vi "test Add-Find-Remove Custom Device.vi"(8 "error in":errorcluster, 11 "TestCase in":refnum<class "Scripting.lvclass">) -> (0 "error out":errorcluster, 3 "TestCase out":refnum<class "Scripting.lvclass">)   [LabVIEW 2020, in "Scripting.lvclass"]
uses:
  Scripting.lvclass
  C:/dev/git/niveristand-custom-device-testing-tools/VeriStandScriptingTestCase/VeriStandScriptingTestCase.lvclass
  niveristand-custom-device-testing-tools/VeriStandScriptingTestCase/VeriStandScriptingTestCase.lvclass/VeriStandScriptingTestCase.ctl
  niveristand-custom-device-testing-tools/VeriStandScriptingTestCase/Read Target.vi
  NationalInstruments.VeriStand.SystemDefinitionAPI
  <vilib>/addons/_JKI Toolkits/VI Tester/TestCase.llb/TestCase.lvclass
  Scripting/AIM MIL-STD-1553 Scripting.lvlib
  C:/Program Files (x86)/National Instruments/LabVIEW 2020/vi.lib/addons/_JKI Toolkits/VI Tester/TestCase.llb/TestCase.lvclass
  C:/dev/git/niveristand-aim-milStd1553-custom-device/Source/Custom Device Support/Tests/Unit/Scripting/Scripting.lvclass
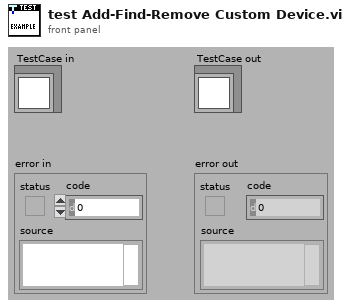
[diagram p1: front panel]
types:
  T1 = typedef "Custom Device API.lvlib/Custom Device Item Ref.ctl" = u64
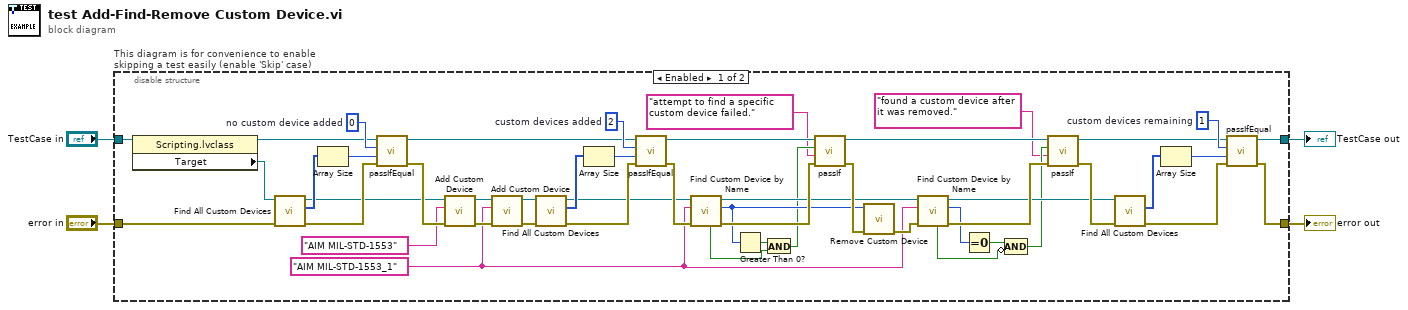
[diagram p0: block diagram]
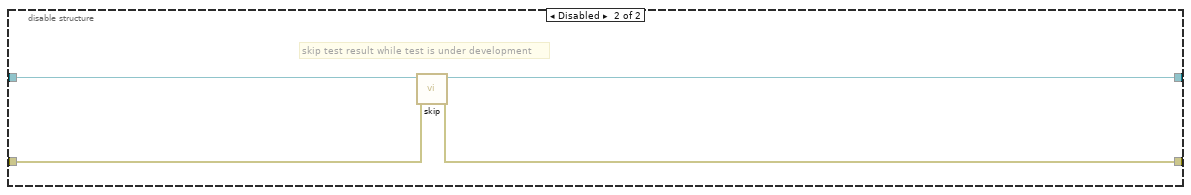
[diagram p2: hidden frame]
diagram:
  n1 = disable-structure "This diagram is for convenience to enable skipping a test easily (enable 'Skip' case)" shown="Enabled" {
    disable-tunnel: "TestCase in" -> [w20 w57]
    disable-tunnel: [w23 w55] -> w1
    disable-tunnel: [w22 w56] -> w3
    disable-tunnel: "error in" -> [w53 w54]
    frame Enabled {
      w7 = "AIM MIL-STD-1553_1" ("name")
      w27 = 1  # custom devices remaining
      w43 = 2  # custom devices added
      w50 = 0  # no custom device added
      n2 = property class="Scripting.lvclass"(reference=w20) -> (reference out=w18:refnum<class "Scripting.lvclass">, "Target"=w19:refnum<k24>)  [unwired: 1 in, 1 out]
      n3 = call "Find All Custom Devices.vi"("error in"=w53, "target"=w19) -> ("error out"=w49:errorcluster, "custom device refs"=w52:T1[], "target out"=w47:refnum<k24>)  [unwired: 7 in]
      n4 = Array Size(array=w52) -> (size(s)=w51:i32)
      n5 = call-dynamic "passIfEqual.vi"("error in (no error)"=w49, "y"=w51, "x"=w50, "TestCase in"=w18) -> ("error out"=w48:errorcluster, "TestCase out"=w17:refnum<class "Scripting.lvclass">)  [unwired: 6 in]
      n6 = call "Add Custom Device.vi"("error in"=w48, "custom device name"="AIM MIL-STD-1553" ("name"), "target"=w47) -> ("error out"=w16:errorcluster, "target out"=w46:refnum<k24>)  [unwired: 6 in, 1 out]
      n7 = call "Add Custom Device.vi"("error in"=w16, "custom device name"=w7, "target"=w46) -> ("error out"=w45:errorcluster, "target out"=w44:refnum<k24>)  [unwired: 6 in, 1 out]
      n8 = call "Find All Custom Devices.vi"("error in"=w45, "target"=w44) -> ("error out"=w40:errorcluster, "custom device refs"=w41:T1[], "target out"=w38:refnum<k24>)  [unwired: 7 in]
      n9 = Array Size(array=w41) -> (size(s)=w42:i32)
      n10 = call-dynamic "passIfEqual.vi"("error in (no error)"=w40, "y"=w42, "x"=w43, "TestCase in"=w17) -> ("error out"=w39:errorcluster, "TestCase out"=w37:refnum<class "Scripting.lvclass">)  [unwired: 6 in]
      n11 = call "Find Custom Device by Name.vi"("error in"=w39, "custom device name"=w7, "target"=w38) -> ("error out"=w36:errorcluster, "custom device ref"=w14:T1, "target out"=w32:refnum<k24>, "found?"=w11:bool)  [unwired: 5 in]
      n12 = Greater Than 0?(x=w14) -> (x > 0?=w15:bool)
      n13 = And(x=w15, y=w11) -> (x .and. y?=w12:bool)
      n14 = call-dynamic "passIf.vi"("error in (no error)"=w36, "message (\"\")"="attempt to find a specific custom device failed." ("message (\"\")"), "pass"=w12, "TestCase in"=w37) -> ("error out"=w35:errorcluster, "TestCase out"=w31:refnum<class "Scripting.lvclass">)  [unwired: 6 in]
      n15 = call "Remove Custom Device.vi"("error in"=w35, "Ballard MIL-STD 1553 custom device"=w14) -> ("error out"=w34:errorcluster)  [unwired: 9 in]
      n16 = call "Find Custom Device by Name.vi"("error in"=w34, "custom device name"=w7, "target"=w32) -> ("error out"=w30:errorcluster, "custom device ref"=w13:T1, "target out"=w28:refnum<k24>, "found?"=w10:bool)  [unwired: 5 in]
      n17 = Equal To 0?(x=w13) -> (x = 0?=w9:bool)
      n18 = Compound Arithmetic op=AND(w9, invert w10) -> (w8:bool)
      n19 = call-dynamic "passIf.vi"("error in (no error)"=w30, "message (\"\")"="found a custom device after it was removed." ("message (\"\")"), "pass"=w8, "TestCase in"=w31) -> ("error out"=w29:errorcluster, "TestCase out"=w26:refnum<class "Scripting.lvclass">)  [unwired: 6 in]
      n20 = call "Find All Custom Devices.vi"("error in"=w29, "target"=w28) -> ("error out"=w25:errorcluster, "custom device refs"=w24:T1[])  [unwired: 7 in, 1 out]
      n21 = Array Size(array=w24) -> (size(s)=w21:i32)
      n22 = call-dynamic "passIfEqual.vi"("error in (no error)"=w25, "y"=w21, "x"=w27, "TestCase in"=w26) -> ("error out"=w22:errorcluster, "TestCase out"=w23:refnum<class "Scripting.lvclass">)  [unwired: 6 in]
    }
    frame Disabled {
      # "skip test result while test is under development"
      n23 = call <vilib>:"skip.vi"("error in (no error)"=w54, "TestCase in"=w57) -> ("error out"=w56:errorcluster, "TestCase out"=w55:refnum<class "Scripting.lvclass">)  [unwired: 8 in]
    }
  }
  "error out" <- w3
  "TestCase out" <- w1
